vi "FGV for result.vi"(8 "Seq id in":i32, 10 "In Data":string[][](array[string]), 11 "Enum":enum16{"Ini", "Write", "Read"}(ring)=enum."Read") -> (0 "Seq id out":i32, 3 "Out Data":string[][](array[string]))   [LabVIEW 2020]
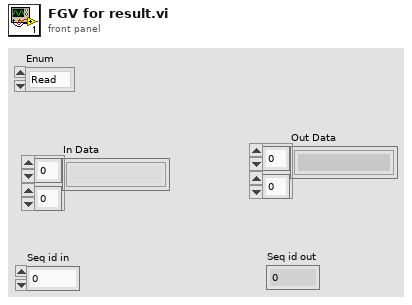
[diagram p1: front panel]
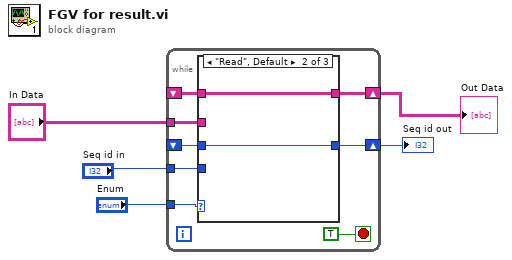
[diagram p0: block diagram]
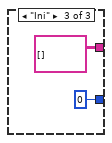
[diagram p3: hidden frame]
diagram:
  n1 = while {
    tunnel: "Enum" -> [w12]
    shift-right: [w6] -> w2
    shift-left: _ -> [w11]
    tunnel: "In Data" -> [w10]
    shift-right: [w8] -> w1
    shift-left: _ -> [w7]
    tunnel: "Seq id in" -> [w9]
    stop <- TRUE stop-if-true
    n2 = case shown="\"Read\", Default" w12 {
      tunnel: w11 -> [_ w16 _]
      tunnel: w10 -> [w14 _ _]
      tunnel: w7 -> [_ w17 _]
      tunnel: [w15 w17 0 ("Numeric")] -> w8
      tunnel: w9 -> [w15 _ _]
      tunnel: [w14 w16 string[][] [] ("In Data")] -> w6
      frame "Write" {
      }
      frame "Read", Default {
      }
      frame "Ini" {
      }
    }
  }
  "Seq id out" <- w1
  "Out Data" <- w2
